vi "DB2.TestLauncher.vi"() -> ()   [LabVIEW 2022 SP3, in "DB2.lvclass"]
uses:
  DB2.lvclass
  Typedefs/DB2 State--enum.ctl
  <vilib>/JKI/JKI SMO/SMO/Typedefs/SMOState --Enum.ctl
  C:/Program Files (x86)/National Instruments/LabVIEW 2022/vi.lib/JKI/JKI SMO/SMO/SMO.lvclass
  <vilib>/JKI/JKI SMO/SMO/SMO.lvclass/SMO.ctl
  <vilib>/JKI/JKI SMO/SMO/Private/ReftoDVR--SMO.vi
  DB2.lvclass/DB2.ctl
  <vilib>/JKI/JKI SMO/SMO/SMO.lvclass
  C:/Users/uib01493/Documents/CIS_580_Data_Analytics_in_SW_Eng/002_Source_Code/002_GUI/002_SRC/DB2/DB2.lvclass
panel:
  in  "Request":bool
  out "Source Code to Directory":path
  out "Report Generation Save Path":path
  out "Requirements Directory":path
  out "SMO State":T1
  in  "Embed?":bool=TRUE
  out "UI State":T2
  out "error out":errorcluster
  in  "Stop":bool
  # "SMO.UI_Embedded Test Launcher"
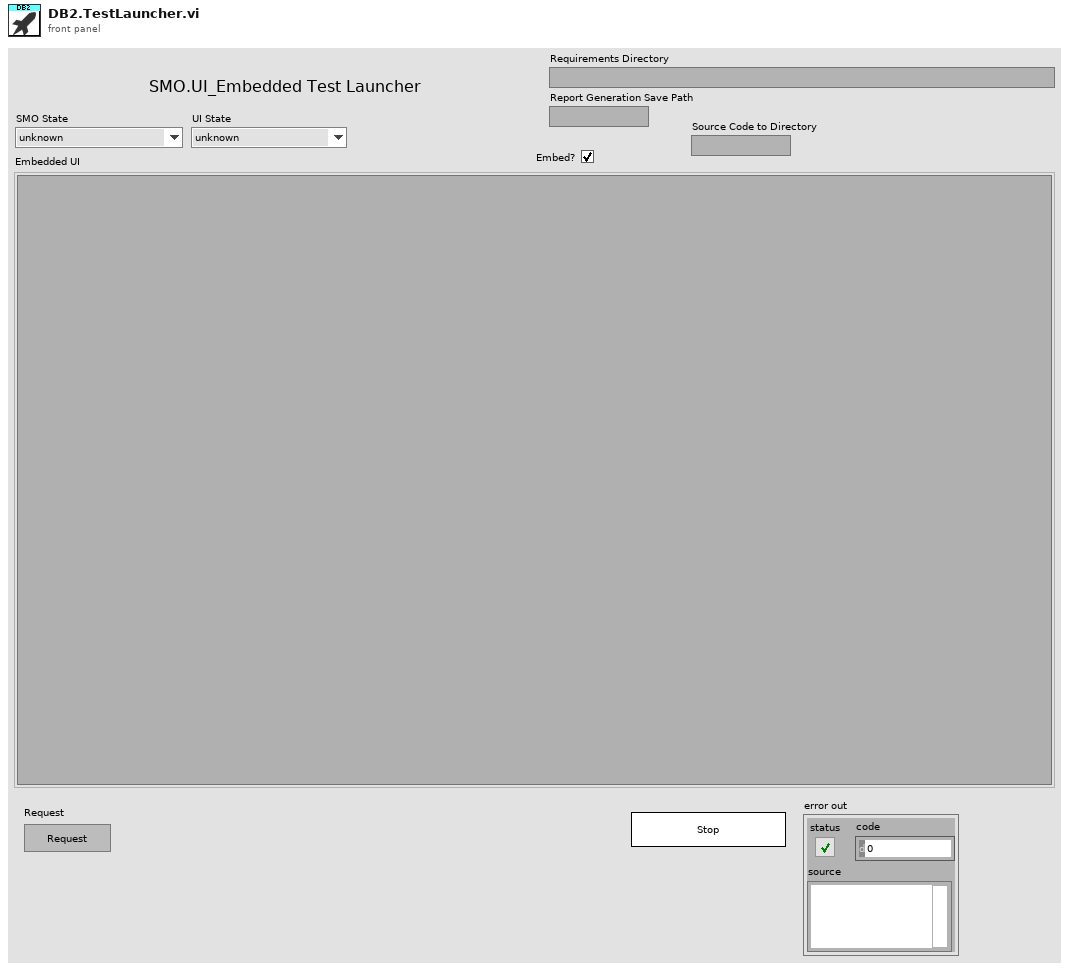
[diagram p1: front panel]
types:
  T1 = typedef "SMO.lvclass/SMOState --Enum.ctl" = enum16{"unknown", "Created", "Started", "Stopped"}
  T2 = typedef "DB2.lvclass/DB2 State--enum.ctl" = enum16{"unknown", "Opened", "Embedded", "Closed"}
  T3 = typedef "SMO.lvclass/Public Events.ctl" = cluster{"Error":refnum<user-event>, "State":refnum<user-event>, "Reserve State":refnum<user-event>}
  T4 = typedef "DB2.lvclass/PublicEvents--Cluster.ctl" = cluster{"UI State":refnum<user-event>, "NewSettingsConfig":refnum<user-event>}
  T5 = cluster{"Event Registration Refnum":refnum<event-registration>}
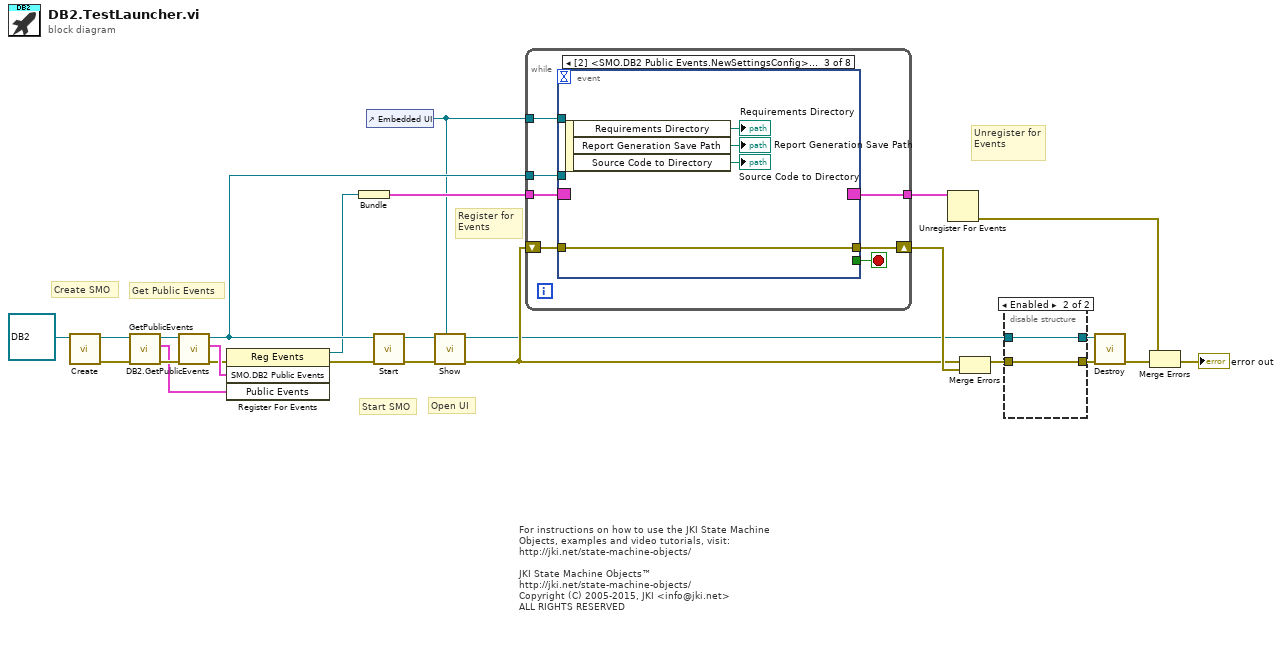
[diagram p0: block diagram]
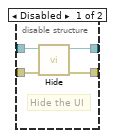
[diagram p2: hidden frame]
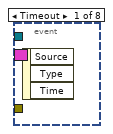
[diagram p3: hidden frame]
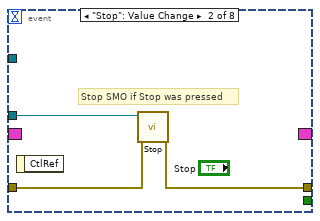
[diagram p4: hidden frame]
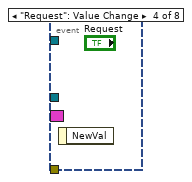
[diagram p5: hidden frame]
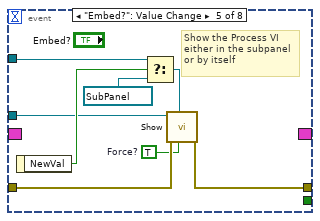
[diagram p6: hidden frame]
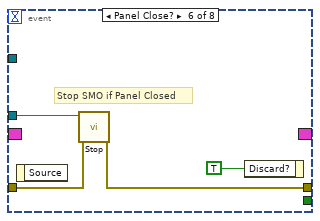
[diagram p7: hidden frame]
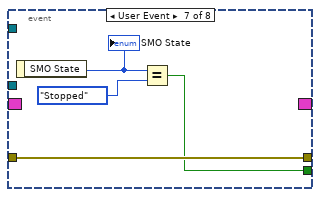
[diagram p8: hidden frame]
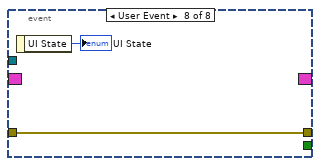
[diagram p9: hidden frame]
diagram:
  # "For instructions on how to use the JKI State Machine Objects, examples and video tutorials, visit:\nhttp://jki.net/state-machine-objects/\n\nJKI State Machine Objects™\nhttp://jki.net/state-machine-objects/\nCopyright (C) 2005-2015, JKI <info@jki.net>\nALL RIGHTS RESERVED"
  # "Get Public Events"
  # "Start SMO"
  # "Create SMO"
  # "Open UI"
  # "Unregister for Events"
  # "Register for Events"
  n1 = call <vilib>:"Create.vi"("SMO"=refnum<class "DB2.lvclass"> refnum ("SMO.UI.lvclass")) -> ("error out"=w13:errorcluster, "SMO out"=w11:refnum<class "DB2.lvclass">)  [unwired: 8 in, 1 out]
  n2 = call <vilib>:"GetPublicEvents.vi"("error in (no error)"=w13, "SMO"=w11) -> ("error out"=w12:errorcluster, "Public Events"=w9:T3, "SMO out"=w10:refnum<class "DB2.lvclass">)  [unwired: 7 in]
  n3 = call "DB2.GetPublicEvents.vi"("error in (no error)"=w12, "DB2"=w10) -> ("error out"=w15:errorcluster, "SMO.DB2 Public Events"=w17:T4, "DB2 out"=w18:refnum<class "DB2.lvclass">)  [unwired: 7 in]
  n4 = register-events(error in=w15, w17, w9) -> (reference out=w16:refnum<event-registration>, error out=w14:errorcluster)  [unwired: 1 in]
  n5 = Bundle("Event Registration Refnum"=w16) -> (w24:T5)  [unwired: 1 in]
  n6 = control-ref of="Embedded UI"() -> (w5:refnum<vi>)
  n7 = call <vilib>:"Start.vi"("error in (no error)"=w14, "SMO"=w18) -> ("error out"=w7:errorcluster, "SMO out"=w8:refnum<class "DB2.lvclass">)  [unwired: 8 in]
  n8 = call "Show.vi"("Subpanel Ref (empty: open detached)"=w5, "error in (no error)"=w7, "DB2"=w8) -> ("error out"=w6:errorcluster, "DB2 out"=w4:refnum<class "DB2.lvclass">)  [unwired: 7 in]
  n9 = while {
    shift-right: [w31] -> w22
    shift-left: w6 -> [w30]
    tunnel: w24 -> [w29]
    tunnel: [w28] -> w25
    tunnel: w18 -> [w27]
    tunnel: w5 -> [w26]
    stop <- w32 stop-if-true
    n10 = event shown="[2] <SMO.DB2 Public Events.NewSettingsConfig>: User Event" {
      selector: w29 -> [_ _ _ _ _ _ _ _]
      dyn-events: [_ _ _ _ _ _ _ _] -> w28
      timeout: _ -> [_ _ _ _ _ _ _ _]
      tunnel: [_ _ _ _ _ _ w52 _] -> w32
      tunnel: w27 -> [_ w33 _ _ w42 w51 _ _]
      tunnel: [_ w35 w39 _ w47 w50 w53 w57] -> w31
      tunnel: w30 -> [_ w34 w39 _ w41 w49 w53 w57]
      tunnel: w26 -> [_ _ _ _ w45 _ _ _]
      event Timeout {
        n11 = event-data() -> ()  [unwired: 1 in, 3 out]
      }
      event "Stop": Value Change {
        # "Stop SMO if Stop was pressed"
        n12 = event-data() -> ()  [unwired: 1 in, 1 out]
        n13 = call <vilib>:"Stop.vi"("error in (no error)"=w34, "SMO"=w33) -> ("error out"=w35:errorcluster)  [unwired: 8 in, 1 out]
      }
      event User Event {
        n14 = event-data() -> ("Requirements Directory"=→"Requirements Directory":path, "Report Generation Save Path"=→"Report Generation Save Path":path, "Source Code to Directory"=→"Source Code to Directory":path)  [unwired: 1 in]
      }
      event "Request": Value Change {
        n15 = event-data() -> ()  [unwired: 1 in, 1 out]
      }
      event "Embed?": Value Change {
        w40 = TRUE  # Force?
        # "Show the Process VI\neither in the subpanel\nor by itself"
        n16 = event-data() -> ("NewVal"=w46:bool)  [unwired: 1 in]
        n17 = Select(t=w45, s=w46, f=refnum<vi> refnum) -> (s? t:f=w44:refnum<vi>)
        n18 = call "Show.vi"("Force? (true)"=w40, "Subpanel Ref (empty: open detached)"=w44, "error in (no error)"=w41, "DB2"=w42) -> ("error out"=w47:errorcluster)  [unwired: 6 in, 1 out]
      }
      event Panel Close? {
        # "Stop SMO if Panel Closed"
        n19 = event-data() -> ()  [unwired: 1 in, 1 out]
        n20 = call <vilib>:"Stop.vi"("error in (no error)"=w49, "SMO"=w51) -> ("error out"=w50:errorcluster)  [unwired: 8 in, 1 out]
        n21 = event-data("Discard?"=TRUE ("OK")) -> ()  [unwired: 1 in, 1 out]
      }
      event User Event {
        n22 = event-data() -> ("SMO State"=w55:T1)  [unwired: 1 in]
        "SMO State" <- w55
        n23 = Equal?(x=w55, y=SMOState_--Enum."Stopped") -> (x = y?=w52:bool)
      }
      event User Event {
        n24 = event-data() -> ("UI State"=→"UI State":T2)  [unwired: 1 in]
      }
    }
  }
  n25 = Unregister For Events(event registration refnum=w25) -> (error out=w21:errorcluster)  [unwired: 1 in]
  n26 = Merge Errors(w6, w22) -> (w2:errorcluster)
  n27 = disable-structure shown="Enabled" {
    disable-tunnel: w4 -> [w61 w63]
    disable-tunnel: [w60 w63] -> w3
    disable-tunnel: w2 -> [w59 w62]
    disable-tunnel: [w58 w62] -> w1
    frame Disabled {
      # "Hide the UI"
      n28 = call "Hide.vi"("error in (no error)"=w59, "DB2"=w61) -> ("error out"=w58:errorcluster, "DB2 out"=w60:refnum<class "DB2.lvclass">)  [unwired: 8 in]
    }
    frame Enabled {
    }
  }
  n29 = call <vilib>:"Destroy.vi"("error in (no error)"=w1, "SMO"=w3) -> ("error out"=w19:errorcluster)  [unwired: 9 in]
  n30 = Merge Errors(w21, w19) -> (→"error out":errorcluster)
